vi "IterateCluster.vi"(0 "Ctl Refnum in":refnum<vi>, 5 "ControlDoBase in":refnum<class "ControlDoBase.lvclass">, 7 "Control Path":string[](array[string]), 11 "error in (no error)":errorcluster) -> (4 "Ctl Refnum out":refnum<vi>, 6 "ControlDoBase out":refnum<class "ControlDoBase.lvclass">, 15 "error out":errorcluster)   [LabVIEW 2016, in "VI.lvlib"]
uses:
  VI.lvlib
  ControlAction/DoBase/ControlDoBase.lvclass
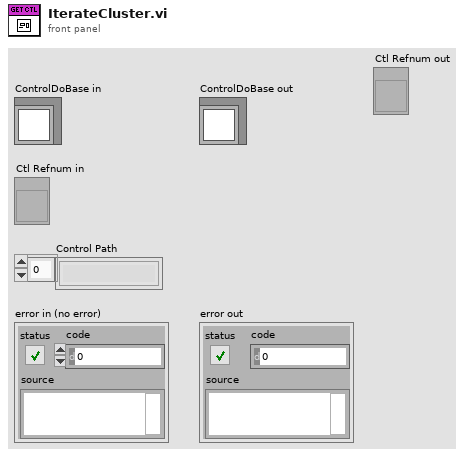
[diagram p1: front panel]
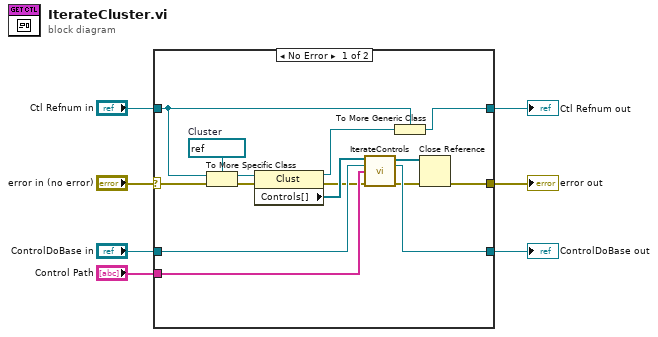
[diagram p0: block diagram]
diagram:
  n1 = case shown="No Error" "error in (no error)" {
    selector: "error in (no error)" -> [w14 w25]
    tunnel: "Control Path" -> [w22 _]
    tunnel: [w21 w23] -> w6
    tunnel: "ControlDoBase in" -> [w20 w23]
    tunnel: [w18 w25] -> w4
    tunnel: [w9 w24] -> w1
    tunnel: "Ctl Refnum in" -> [w8 w24]
    frame No Error {
      w11 = refnum<vi> refnum  # Cluster
      n2 = To More Specific Class(target class=w11, reference=w8, error in=w14) -> (specific class reference=w12:refnum<vi>, error out=w13:errorcluster)
      n3 = property class="Clust"(reference=w12, error in=w13) -> (reference out=w16:refnum<vi>, error out=w15:errorcluster, "Controls[]"=w17:refnum<vi>[])
      n4 = call "IterateControls.vi"("Controls[] In"=w17, "ControlDoBase in"=w20, "Control Path"=w22, "error in (no error)"=w15) -> ("Controls[] Out"=w19:refnum<vi>[], "ControlDoBase out"=w21:refnum<class "ControlDoBase.lvclass">, "error out"=w10:errorcluster)  [unwired: 9 in]
      n5 = To More Generic Class(target class=w8, reference=w16) -> (generic class reference=w9:refnum<vi>)
      n6 = Close Reference(reference=w19, error in (no error)=w10) -> (error out=w18:errorcluster)
    }
    frame Error {
    }
  }
  "ControlDoBase out" <- w6
  "error out" <- w4
  "Ctl Refnum out" <- w1
